vi "SetUnits.vi"(7 "Timeout (ms)":u32=2000, 8 "Error In":errorcluster, 10 "Units":T1, 11 "Sierra M100 In":refnum<visa-resource-name>) -> (0 "Error Out":errorcluster, 2 "Set?":bool, 3 "Sierra M100 Out":refnum<visa-resource-name>)   [LabVIEW 2012, in "Sierra-M100.lvlib"]
doc: "This VI sets the units of measure for the flow rate. This includes the units for the setpoint and reading."
uses:
  Sierra-M100.lvlib
  Controls/Units.ctl
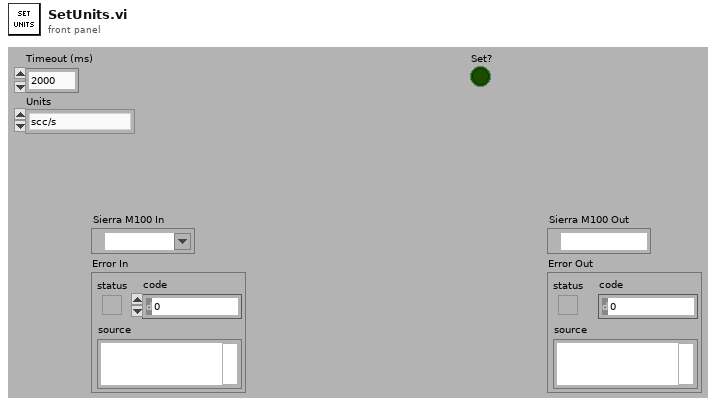
[diagram p1: front panel]
types:
  T1 = typedef "Sierra-M100.lvlib/Units.ctl" = enum16{"scc/s", "scc/m", "scc/H", "Ncc/s", "Ncc/m", "Ncc/H", "SCF/s", "SCF/m", "SCF/H", "NM3/s", "NM3/m", "NM3/H", "SM3/s", "SM3/m", "SM3/H", "sl/s", "sl/m", "sl/H", "NL/s", "NL/m", "Nl/H", "g/s", "g/m", "g/H", "kg/s", "kg/m", "kg/H", "lb/s", "lb/m", "lb/H"}
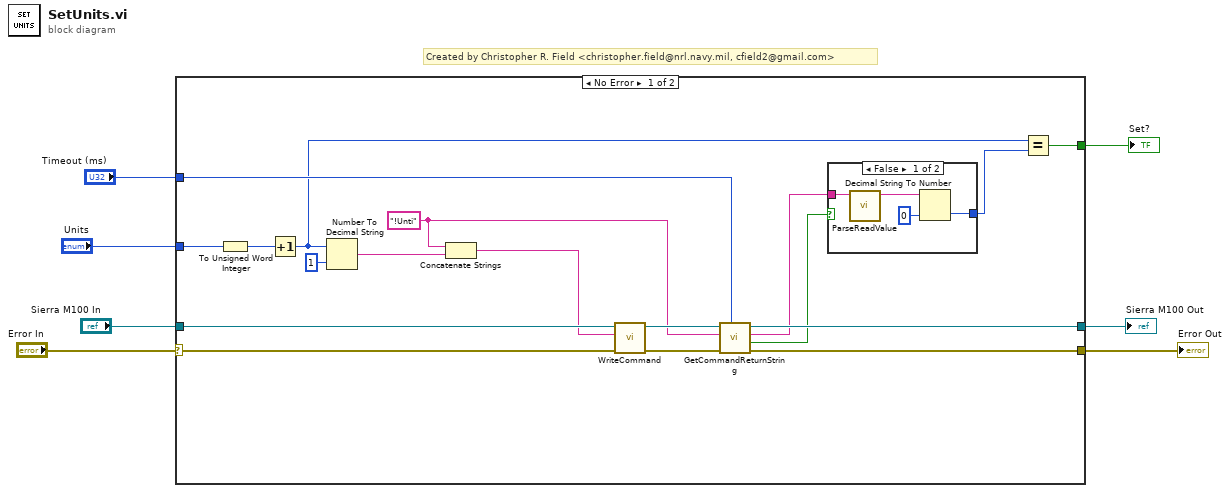
[diagram p0: block diagram]
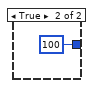
[diagram p2: hidden frame]
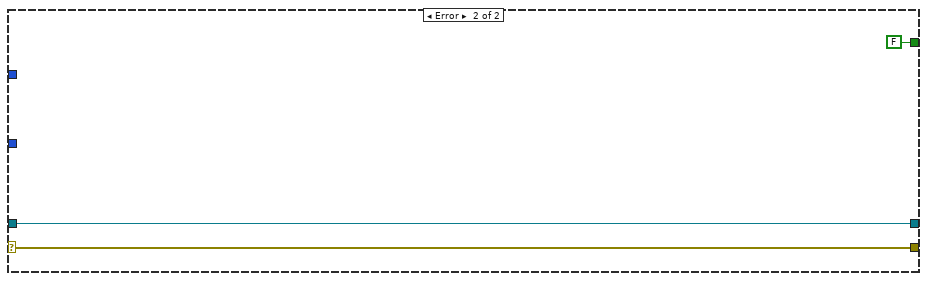
[diagram p3: hidden frame]
diagram:
  # "Created by Christopher R. Field <christopher.field@nrl.navy.mil, cfield2@gmail.com>"
  n1 = case shown="No Error" "Error In" {
    selector: "Error In" -> [w8 w32]
    tunnel: [w20 w33] -> w7
    tunnel: [w19 w32] -> w6
    tunnel: "Sierra M100 In" -> [w18 w33]
    tunnel: "Timeout (ms)" -> [w15 _]
    tunnel: [w10 FALSE] -> w3
    tunnel: "Units" -> [w9 _]
    frame No Error {
      w16 = "!Unti"
      n2 = To Unsigned Word Integer(number=w9) -> (unsigned 16bit integer=w25:u16)
      n3 = Increment(x=w25) -> (x+1=w11:u16)
      n4 = Number To Decimal String(number=w11, width (-)=i16 1) -> (decimal integer string=w23:string)
      n5 = Concatenate Strings(w16, w23) -> (w17:string)
      n6 = call "WriteCommand.vi"("Error In"=w8, "Command"=w17, "Smart Trak 2 In"=w18) -> ("Error Out"=w21:errorcluster, "Smart Trak 2 Out"=w22:refnum<visa-resource-name>)  [unwired: 5 in, 2 out]
      n7 = call "GetCommandReturnString.vi"("Timeout (ms)"=w15, "Error In"=w21, "Command"=w16, "Smart Trak 2 In"=w22) -> ("Error Out"=w19:errorcluster, "Timeout?"=w14:bool, "Return String"=w13:string, "Smart Trak 2 Out"=w20:refnum<visa-resource-name>)  [unwired: 4 in]
      n8 = case shown="False" w14 {
        tunnel: w13 -> [w29 _]
        tunnel: [w26 u16 100] -> w12
        frame False {
          n9 = call "ParseReadValue.vi"("Read Buffer"=w29) -> ("Value"=w28:string)  [unwired: 10 in]
          n10 = Decimal String To Number(string=w28, default (0L)=u16 0 ("default (0 I32)")) -> (number=w26:u16)  [unwired: 1 in, 1 out]
        }
        frame True {
        }
      }
      n11 = Equal?(x=w11, y=w12) -> (x = y?=w10:bool)
    }
    frame Error {
    }
  }
  "Sierra M100 Out" <- w7
  "Error Out" <- w6
  "Set?" <- w3
